vi "Set Report Orientation.vi"(0 "report in":refnum<class "NI_Standard Report.lvclass">, 5 "orientation (portrait)":i32(ring) items=["portrait", "landscape"], 11 "error in (no error)":errorcluster) -> (4 "report out":refnum<class "NI_Standard Report.lvclass">, 15 "error out":errorcluster)   [LabVIEW 2020, in "NI_Standard Report.lvclass"]
doc: "Determines whether the report is printed in landscape or portrait orientation."
uses:
  NI_Standard Report.lvclass
panel:
  in  "warning msg":string="Setting the orientation of a Standard Report to 'landscape' is no longer supported."
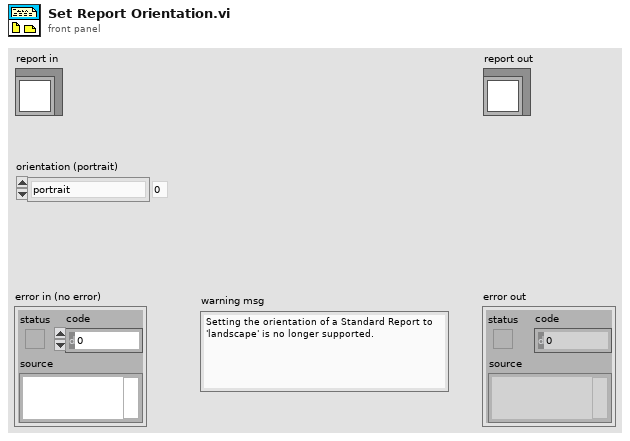
[diagram p1: front panel]
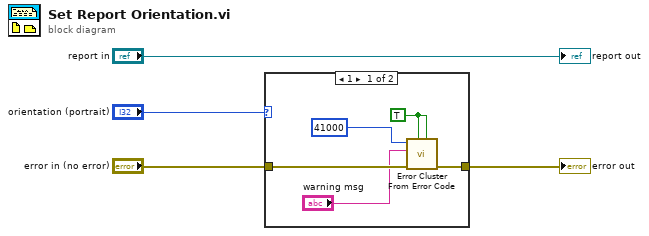
[diagram p0: block diagram]
diagram:
  n1 = case shown="1" "orientation (portrait)" {
    tunnel: "error in (no error)" -> [w8 w10]
    tunnel: [w9 w10] -> w1
    frame 1 {
      w6 = TRUE ("is warning? (False)")
      n2 = call "Error Cluster From Error Code.vi"("is warning? (False)"=w6, "show call chain? (False)"=w6, "error in (no error)"=w8, "error message (\"\")"="warning msg", "error code (0)"=41000) -> ("error out"=w9:errorcluster)  [unwired: 4 in]
    }
    frame Default {
    }
  }
  "error out" <- w1
  "report out" <- "report in"
